vi "Event Handle Loop_Draw Picture.vi"(8 "error in (no error)":errorcluster, 10 "Picture":picture, 11 "QMenu Class in":refnum<class "QMenu Class.lvclass">) -> (0 "error out":errorcluster, 3 "QMenu Class out":refnum<class "QMenu Class.lvclass">)   [LabVIEW 2020, in "QTab.lvlib" / "QMenu Class.lvclass"]
uses:
  QMenu Class.lvclass
  QMenu Class.lvclass/QMenu Class.ctl
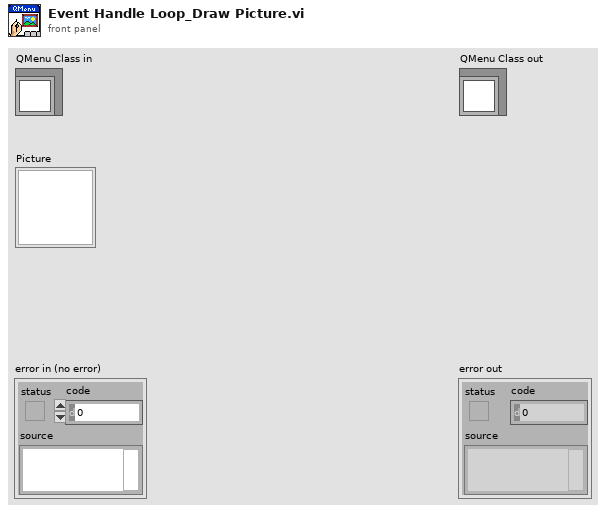
[diagram p1: front panel]
types:
  T1 = typedef "imagedata.ctl" = cluster{"image type":i32, "image depth":i32, "image":u8[], "mask":u8[], "colors":u32[], "Rectangle":cluster{"left":i16, "top":i16, "right":i16, "bottom":i16}}
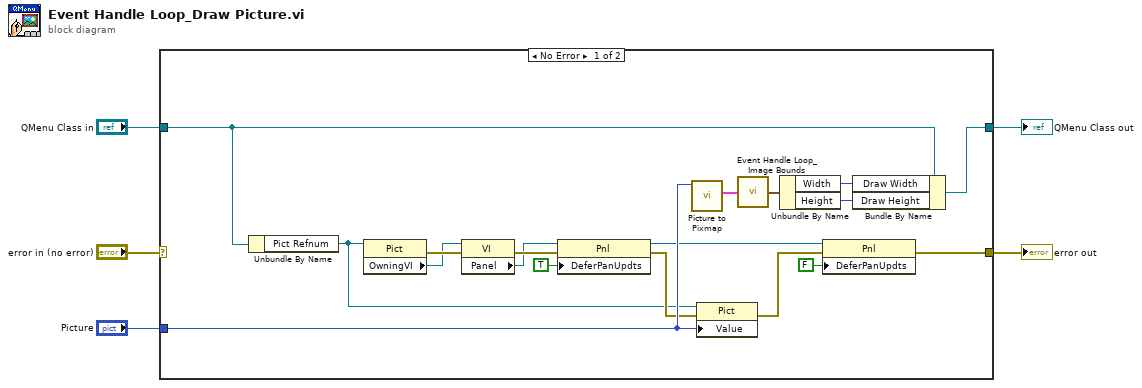
[diagram p0: block diagram]
diagram:
  n1 = case shown="No Error" "error in (no error)" {
    selector: "error in (no error)" -> [_ w25]
    tunnel: "QMenu Class in" -> [w22 w24]
    tunnel: "Picture" -> [w23 _]
    tunnel: [w9 w25] -> w3
    tunnel: [w21 w24] -> w1
    frame No Error {
      n2 = Unbundle By Name(w22) -> ("Pict Refnum"=w6:refnum<vi>)
      n3 = property class="Pict"(reference=w6) -> (error out=w16:errorcluster, "OwningVI"=w15:refnum<vi>)  [unwired: 1 in, 1 out]
      n4 = property class="VI"(reference=w15, error in=w16) -> (error out=w14:errorcluster, "Panel"=w13:refnum<vi>)  [unwired: 1 out]
      n5 = property class="Pnl"(reference=w13, error in=w14, "DeferPanUpdts"=TRUE ("Defer Panel Updates")) -> (reference out=w10:refnum<vi>, error out=w11:errorcluster)
      n6 = call <vilib>:"Picture to Pixmap.vi"("picture"=w23) -> ("image data"=w20:T1)  [unwired: 9 in, 1 out]
      n7 = property class="Pict"(reference=w6, error in=w11, "Value"=w23) -> (error out=w8:errorcluster)  [unwired: 1 out]
      n8 = call "Event Handle Loop_Image Bounds.vi"("Image"=w20) -> ("Bounds"=w19:cluster{"Width":i16, "Height":i16})
      n9 = Unbundle By Name(w19) -> ("Width"=w18:i16, "Height"=w17:i16)
      n10 = property class="Pnl"(reference=w10, error in=w8, "DeferPanUpdts"=FALSE ("Defer Panel Updates")) -> (error out=w9:errorcluster)  [unwired: 1 out]
      n11 = Bundle By Name(cluster=w22, "Draw Width"=w18, "Draw Height"=w17) -> (w21:refnum<class "QMenu Class.lvclass">)
    }
    frame Error {
    }
  }
  "error out" <- w3
  "QMenu Class out" <- w1
